vi "Create Map from Values Indexes to Channel and Label Indexes.vi"(6 "disable channel included in group":bool, 8 "error in":errorcluster, 11 "RT hardware channels":T2[](array[typedef]) {"labels settings for RT"."Label Timestamp Channel Data Reference" format="%.0x"; "labels settings for RT"."Word Initial Raw Value" format="%032.0f"; "labels settings for RT"."Label Disable/Trigger Channel Reference" format="%.0x"; "labels settings for RT"."parameter driver data"."Tx parameter refs" format="%.0x"; "labels settings for RT"."SDI" format="%02b"; "labels settings for RT"."label" format="%.0o"}) -> (0 "error out":errorcluster, 3 "map from values index to RT info indexes":T1)   [LabVIEW 2020, in "AIM ARINC 429 Engine.lvlib" / "Custom Device.lvlib"]
uses:
  Custom Device.lvlib
  Shared/RT Hardware Channel Settings.ctl
  Shared/RT Label Settings.ctl
  Shared/Label.ctl
  Shared/RT Parameters.ctl
  Shared/Parameter Definition.ctl
  <vilib>/NI/NI VeriStand Encoding and Decoding/Encoding.ctl
  <vilib>/NI VeriStand/Custom Device API/Custom Device Item Ref.ctl
  Shared/Transfer Type.ctl
  <vilib>/NI VeriStand/Custom Device API/Data Reference.ctl
  Shared/Map of Values Indexes to Channel and Label Indexes.ctl
  <vilib>/NI/NI VeriStand Encoding and Decoding/Encoding and Decoding.lvlib
  <vilib>/NI VeriStand/Custom Device API/Custom Device API.lvlib
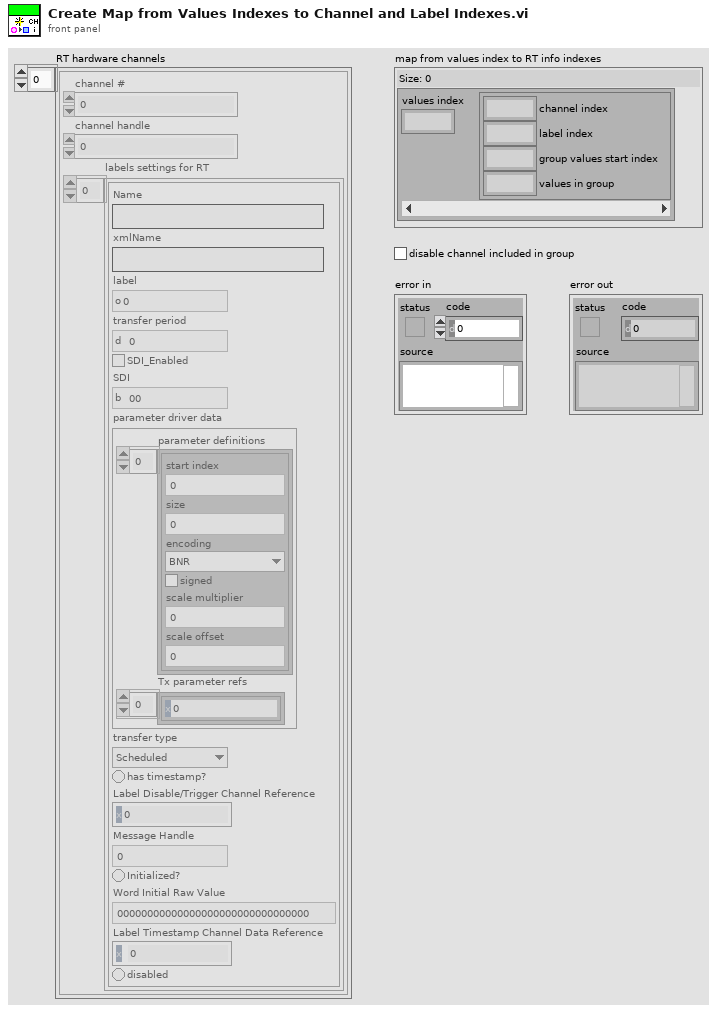
[diagram p1: front panel]
types:
  T1 = typedef "Map of Values Indexes to Channel and Label Indexes.ctl" = map{i32, cluster{"channel index":i32, "label index":i32, "group values start index":i32, "values in group":i32}}
  T2 = typedef "RT Hardware Channel Settings.ctl" = cluster{"channel #":u16, "channel handle":u64, "labels settings for RT":T3[]}
  T3 = typedef "RT Label Settings.ctl" = cluster{"Name":string, "xmlName":string, "label":T4, "transfer period":u32, "SDI_Enabled":bool, "SDI":u8, "parameter driver data":T5, "transfer type":T9, "has timestamp?":bool, "Label Disable/Trigger Channel Reference":T8, "Message Handle":u64, "Initialized?":bool, "Word Initial Raw Value":u32, "Label Timestamp Channel Data Reference":T10, "disabled":bool}
  T4 = typedef "Label.ctl" = u8
  T5 = typedef "RT Parameters.ctl" = cluster{"parameter definitions":T6[], "Tx parameter refs":T8[]}
  T6 = typedef "Parameter Definition.ctl" = cluster{"start index":i32, "size":i32, "encoding":T7, "signed":bool, "scale multiplier":dbl, "scale offset":dbl}
  T7 = typedef "Encoding and Decoding.lvlib/Encoding.ctl" = enum16{"BNR", "BCD", "Discrete"}
  T8 = typedef "Custom Device API.lvlib/Custom Device Item Ref.ctl" = u64
  T9 = typedef "Transfer Type.ctl" = enum16{"Scheduled", "Acyclic", "Block", "Strobe"}
  T10 = typedef "Custom Device API.lvlib/Data Reference.ctl" = i32
  T11 = cluster{"channel index":i32, "label index":i32, "group values start index":i32, "values in group":i32}
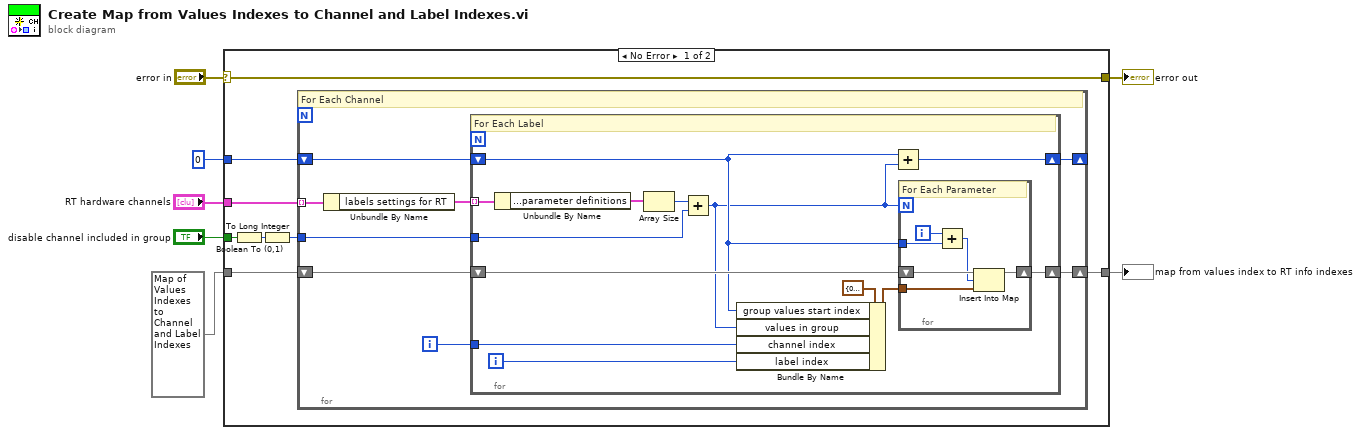
[diagram p0: block diagram]
diagram:
  n1 = case shown="No Error" "error in" {
    selector: "error in" -> [w11 w44]
    tunnel: "RT hardware channels" -> [w15 _]
    tunnel: 0 -> [w14 _]
    tunnel: T1 {} ("map") -> [w13 w43]
    tunnel: [w12 w43] -> w4
    tunnel: [w11 w44] -> w2
    tunnel: "disable channel included in group" -> [w10 _]
    frame No Error {
      n2 = Boolean To (0,1)(Boolean=w10) -> (0, 1=w9:i16)
      n3 = To Long Integer(number=w9) -> (32bit integer=w8:i32)
      n4 = for {
        tunnel: w15 -> [w23] mode=indexing
        shift-right: [w17] -> _
        shift-left: w14 -> [w19]
        shift-right: [w20] -> w12
        shift-left: w13 -> [w21]
        tunnel: w8 -> [w16]
        i -> [w18]
        # "For Each Channel"
        n5 = Unbundle By Name(w23) -> ("labels settings for RT"=w22:T3[])
        n6 = for {
          tunnel: w22 -> [w36] mode=indexing
          shift-right: [w33] -> w20
          shift-left: w21 -> [w34]
          tunnel: w18 -> [w32]
          shift-right: [w28] -> w17
          shift-left: w19 -> [w27]
          tunnel: w16 -> [w24]
          i -> [w31]
          # "For Each Label"
          n7 = Unbundle By Name(w36) -> ("parameter driver data.parameter definitions"=w35:T6[])
          n8 = Array Size(array=w35) -> (size(s)=w26:i32)
          n9 = Add(x=w26, y=w24) -> (x+y=w25:i32)
          n10 = Bundle By Name(cluster=T11 {"channel index"=0, "label index"=0, "group values start index"=0, "values in group"=0} ("value"), "group values start index"=w27, "values in group"=w25, "channel index"=w32, "label index"=w31) -> (w29:T11)
          n11 = Add(x=w27, y=w25) -> (x+y=w28:i32)
          n12 = for {
            N: w25 -> [_]
            shift-right: [w41] -> w33
            shift-left: w34 -> [w42]
            tunnel: w27 -> [w39]
            tunnel: w29 -> [w38]
            i -> [w40]
            # "For Each Parameter"
            n13 = Add(x=w40, y=w39) -> (x+y=w37:i32)
            n14 = Insert Into Map(map in=w42, key=w37, value=w38) -> (map out=w41:T1)  [unwired: 2 out]
          }
        }
      }
    }
    frame Error {
    }
  }
  "map from values index to RT info indexes" <- w4
  "error out" <- w2
